vi "PicoScope2000Stop.vi"(8 "error in (no error)":errorcluster, 11 "handle in":i16) -> (0 "error out":errorcluster, 3 "handle out":i16)   [LabVIEW 2009]
doc: "This stops the device capturing data and should be called before retrieving data from the device."
uses:
  ps2000.dll
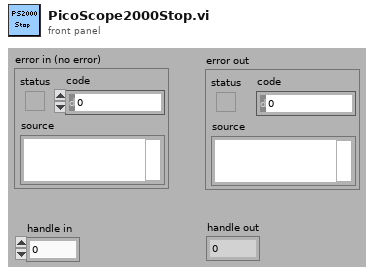
[diagram p1: front panel]
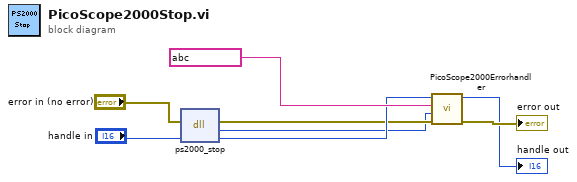
[diagram p0: block diagram]
diagram:
  n1 = dll-call lib="PS2000.dll" fn="ps2000_stop"(error in="error in (no error)", "handle"="handle in") -> (error out=w2:errorcluster, "return"=w1:i16, "handle"=w3:i16)  [unwired: 2 in, 1 out]
  n2 = call "PicoScope2000Errorhandler.vi"("Handle in"=w3, "API function"=string ? ("source"), "Return"=w1, "error in (no error)"=w2) -> ("Handle out"=→"handle out":i16, "error out"=→"error out":errorcluster)  [unwired: 5 in]
